vi "02_PixelShifting.vi"   [LabVIEW 2020]
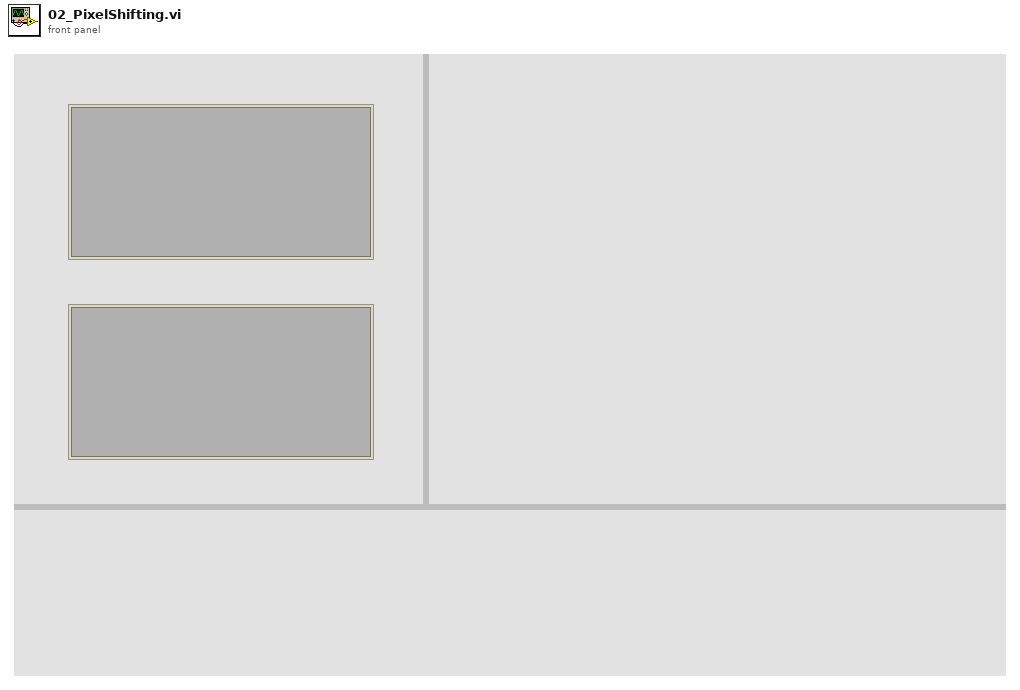
[diagram p1: front panel]
types:
  T1 = typedef "LVRectTypeDef.ctl" = cluster{"Left":i16, "Top":i16, "Right":i16, "Bottom":i16}
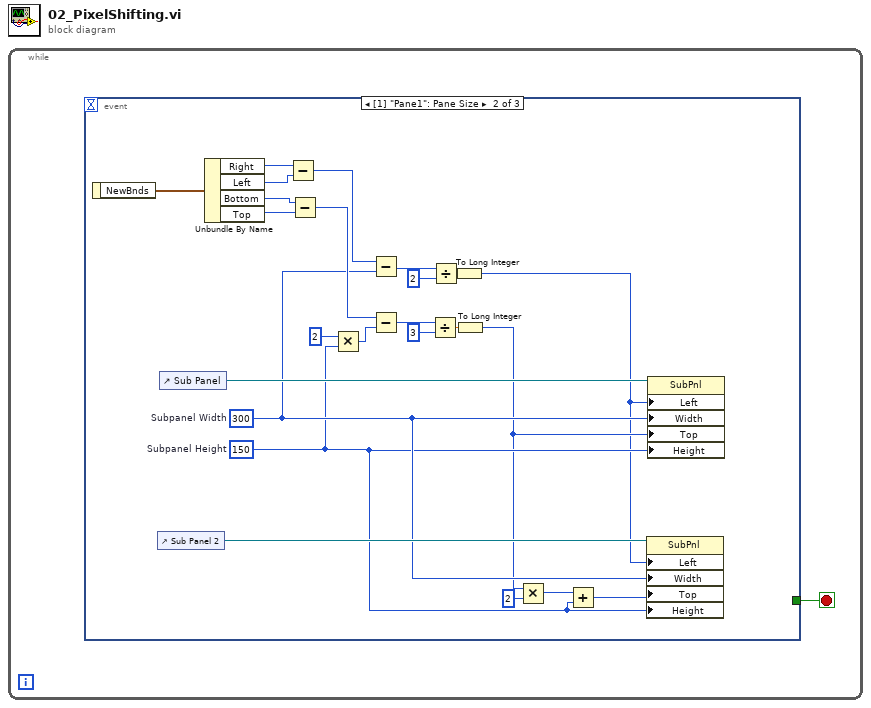
[diagram p0: block diagram]
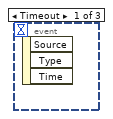
[diagram p2: hidden frame]
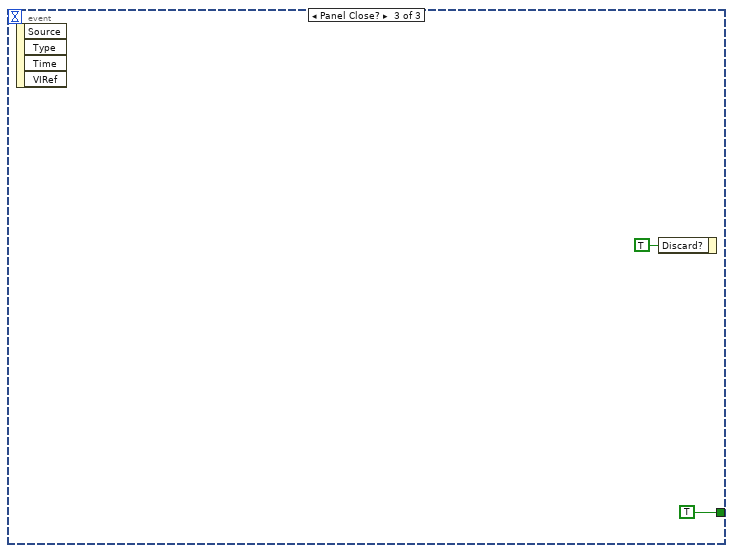
[diagram p3: hidden frame]
diagram:
  n1 = while {
    stop <- w1 stop-if-true
    n2 = event shown="[1] \"Pane1\": Pane Size" {
      selector: _ -> [_ _ _]
      dyn-events: _ -> [_ _ _]
      timeout: _ -> [_ _ _]
      tunnel: [_ _ TRUE] -> w1
      event Timeout {
        n3 = event-data() -> ()  [unwired: 1 in, 3 out]
      }
      event Pane Size {
        w5 = u32 150  # Subpanel Height
        w11 = u32 300  # Subpanel Width
        n4 = event-data() -> ("NewBnds"=w25:T1)  [unwired: 1 in]
        n5 = control-ref of="Sub Panel 2"() -> (w18:refnum<vi>)
        n6 = control-ref of="Sub Panel"() -> (w19:refnum<vi>)
        n7 = Unbundle By Name(w25) -> ("Right"=w24:i16, "Left"=w23:i16, "Bottom"=w22:i16, "Top"=w21:i16)
        n8 = Subtract(x=w24, y=w23) -> (x-y=w12:i16)
        n9 = Subtract(x=w22, y=w21) -> (x-y=w15:i16)
        n10 = Multiply(x=2, y=w5) -> (x*y=w8:u32)
        n11 = Subtract(x=w12, y=w11) -> (x-y=w10:u32)
        n12 = Subtract(x=w15, y=w8) -> (x-y=w9:u32)
        n13 = Divide(x=w9, y=i16 3) -> (x/y=w14:dbl)
        n14 = Divide(x=w10, y=i16 2) -> (x/y=w17:dbl)
        n15 = To Long Integer(number=w17) -> (32bit integer=w2:i32)
        n16 = To Long Integer(number=w14) -> (32bit integer=w3:i32)
        n17 = Multiply(x=w3, y=2) -> (x*y=w6:i32)
        n18 = Add(x=w6, y=w5) -> (x+y=w4:u32)
        n19 = property class="SubPnl"(reference=w18, "Left"=w2, "Width"=w11, "Top"=w4, "Height"=w5) -> ()  [unwired: 1 in, 2 out]
        n20 = property class="SubPnl"(reference=w19, "Left"=w2, "Width"=w11, "Top"=w3, "Height"=w5) -> ()  [unwired: 1 in, 2 out]
      }
      event Panel Close? {
        n21 = event-data() -> ()  [unwired: 1 in, 4 out]
        n22 = event-data("Discard?"=TRUE) -> ()  [unwired: 1 in, 1 out]
      }
    }
  }
